vi "Example1.vi"() -> ()   [LabVIEW 2020, in "LcPictureBox.lvclass"]
uses:
  LcPictureBox.lvclass
  SmoothingMode.ctl
  Pen.ctl
  <vilib>/numeric/Random Number (Range) U64.vi
  <vilib>/numeric/Random Number (Range) DBL.vi
  <vilib>/numeric/sub_Random U32.vi
  System.Windows.Forms
panel:
  in  "PictureBox":refnum<k24>(container)
  in  "Stop":bool
  out "Updating":u32
  out "Drawing":u32
  out "error out":errorcluster
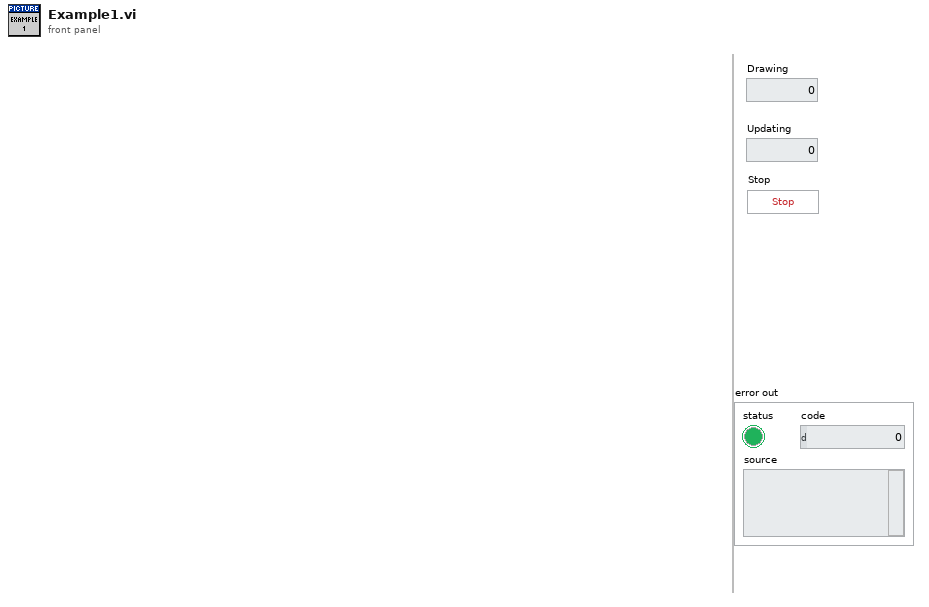
[diagram p1: front panel]
types:
  T1 = typedef "LcPictureBox.lvclass/SmoothingMode.ctl" = enum16{"None", "HighSpeed", "HighQuality", "AntiAlias"}
  T2 = typedef "LcPictureBox.lvclass/Pen.ctl" = cluster{"Width":u16, "Style":enum32{"Solid", "Dash", "Dot", "DashDot", "DashDotDot"}}
  T3 = cluster{"X":sgl, "Y":sgl, "Width":sgl, "Height":sgl}
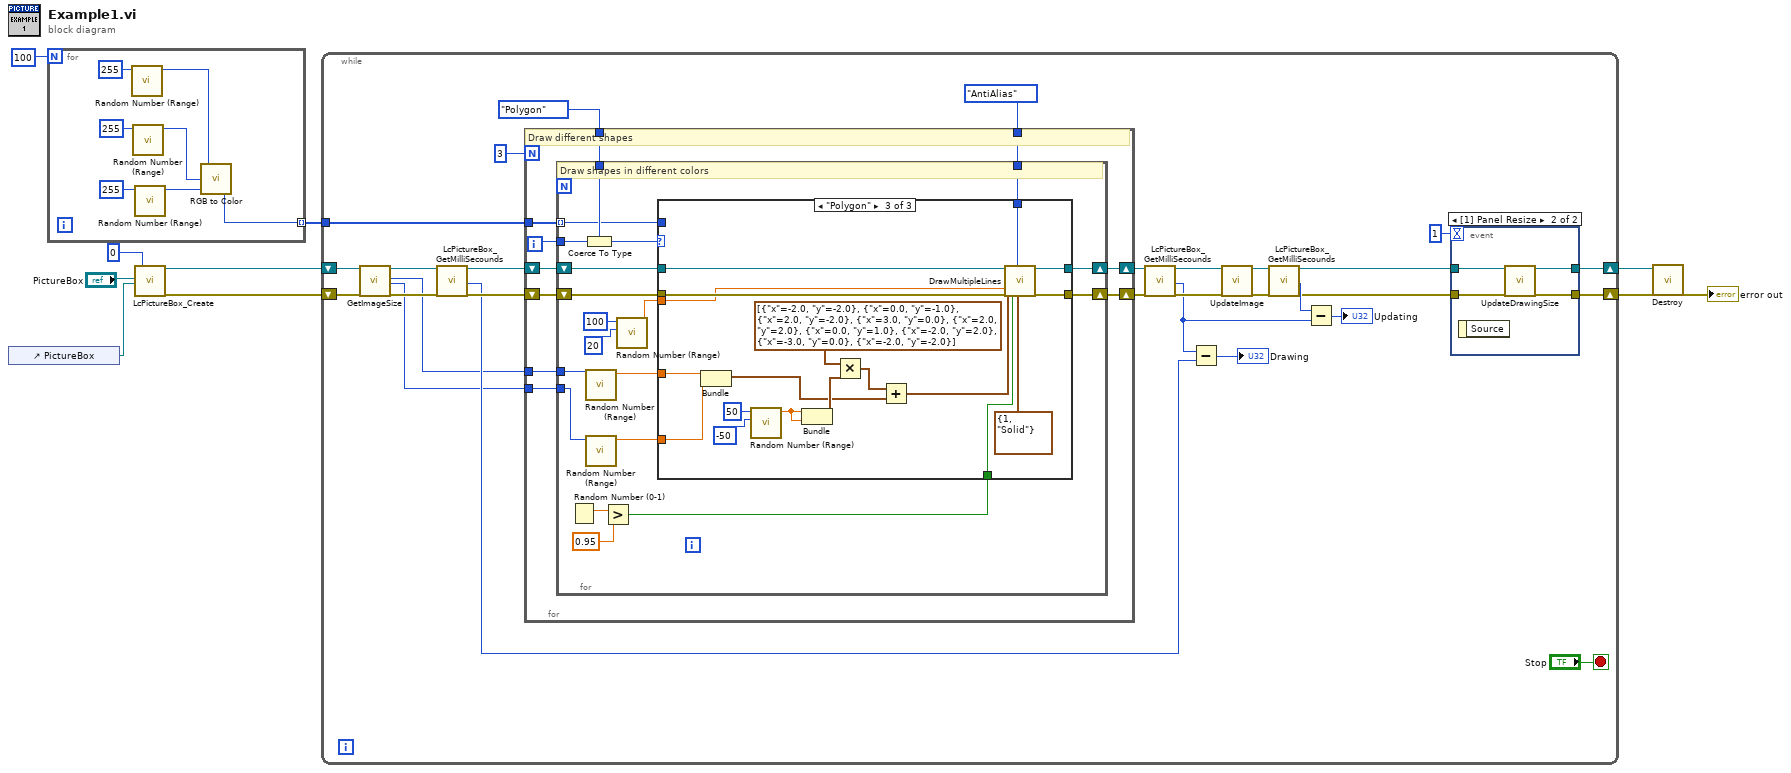
[diagram p0: block diagram]
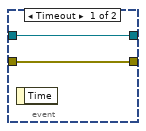
[diagram p2: hidden frame]
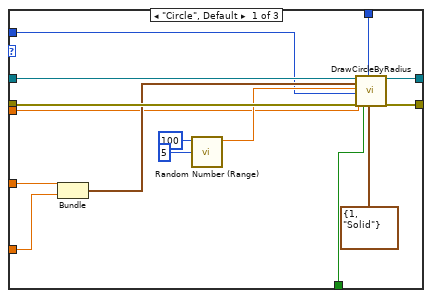
[diagram p3: hidden frame]
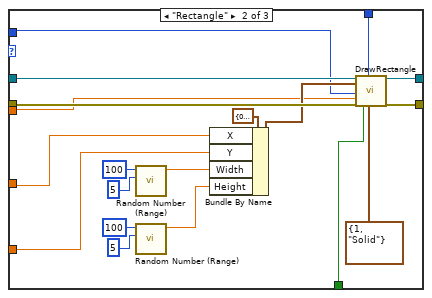
[diagram p4: hidden frame]
diagram:
  n1 = control-ref of="PictureBox"() -> (w2:refnum<vi>)
  n2 = for {
    N: 100 -> [_]
    tunnel: [w11] -> w4 mode=indexing
    n3 = call-poly <vilib>:"Random Number (Range).vi"("upper bound (100)"=u64 255) -> ("number"=w12:u64)  [unwired: 10 in]
    n4 = call-poly <vilib>:"Random Number (Range).vi"("upper bound (100)"=u64 255) -> ("number"=w13:u64)  [unwired: 10 in]
    n5 = call-poly <vilib>:"Random Number (Range).vi"("upper bound (100)"=u64 255) -> ("number"=w15:u64)  [unwired: 10 in]
    n6 = call <vilib>:"RGB to Color.vi"("B"=w15, "G"=w13, "R"=w12) -> ("Color"=w11:u32)
  }
  n7 = call "LcPictureBox_Create.vi"("PictureBox"="PictureBox", "PictureBoxActiveXReference"=w2, "CacheNumberOfPensAndColors(0)"=0 ("CacheNumberOfPensAndColors(1000)")) -> ("reference out"=w7:refnum<class "LcPictureBox.lvclass">, "Error Out"=w6:errorcluster)  [unwired: 14 in, 1 out]
  n8 = while {
    shift-right: [w25] -> w8
    shift-left: w7 -> [w23]
    shift-right: [w24] -> w10
    shift-left: w6 -> [w18]
    tunnel: w4 -> [w30]
    stop <- "Stop" stop-if-true
    n9 = call-dynamic "GetImageSize.vi"("reference in"=w23, "error in (no error)"=w18) -> ("reference out"=w22:refnum<class "LcPictureBox.lvclass">, "Width"=w20:i32, "Height"=w19:i32, "error out"=w21:errorcluster)  [unwired: 14 in]
    n10 = call "LcPictureBox_GetMilliSecounds.vi"("error in (no error)"=w21) -> ("msValue"=w29:u32, "error out"=w42:errorcluster)  [unwired: 17 in]
    n11 = for {
      N: 3 -> [_]
      tunnel: SmoothingMode."AntiAlias" ("SmoothingMode") -> [w55]
      shift-right: [w57] -> w37
      shift-left: w22 -> [w59]
      shift-right: [w58] -> w43
      shift-left: w42 -> [w56]
      tunnel: enum16{"Circle", "Rectangle", "Polygon"}."Polygon" -> [w53]
      tunnel: w20 -> [w52]
      tunnel: w19 -> [w51]
      tunnel: w30 -> [w50]
      i -> [w54]
      # "Draw different shapes"
      n12 = for {
        shift-right: [w75] -> w57
        shift-left: w59 -> [w78]
        shift-right: [w76] -> w58
        shift-left: w56 -> [w77]
        tunnel: w55 -> [w74]
        tunnel: w54 -> [w73]
        tunnel: w53 -> [w71]
        tunnel: w52 -> [w70]
        tunnel: w51 -> [w69]
        tunnel: w50 -> [w63] mode=indexing
        # "Draw shapes in different colors"
        n13 = Random Number (0-1)() -> (number: 0 to 1=w62:dbl)
        n14 = Coerce To Type(0:w73, 1:w71) -> (2:w72:enum16{"Circle", "Rectangle", "Polygon"})
        n15 = call-poly <vilib>:"Random Number (Range).vi"("upper bound (100)"=w70) -> ("number"=w68:dbl)  [unwired: 10 in]
        n16 = call-poly <vilib>:"Random Number (Range).vi"("upper bound (100)"=w69) -> ("number"=w67:dbl)  [unwired: 10 in]
        n17 = Greater?(x=w62, y=0.95) -> (0:w60:bool)
        n18 = call-poly <vilib>:"Random Number (Range).vi"("lower bound (0)"=i64 20 ("lower bound (-100)"), "upper bound (100)"=i64 100) -> ("number"=w64:dbl)  [unwired: 9 in]
        n19 = case shown="\"Polygon\"" w72 {
          tunnel: w78 -> [w93 w112 w130]
          tunnel: w77 -> [w92 w111 w129]
          tunnel: [w91 w110 w128] -> w76
          tunnel: [w90 w109 w127] -> w75
          tunnel: w74 -> [w88 w107 w125]
          tunnel: w68 -> [w87 w104 w124]
          tunnel: w67 -> [w86 w103 w123]
          tunnel: w64 -> [w81 w95 w121]
          tunnel: w63 -> [w80 w96 _]
          tunnel: w60 -> [w79 w94 w120]
          frame "Circle", Default {
            n20 = Bundle("number"=w87, "number"=w86) -> (w85:cluster{"number":dbl, "number":dbl})  [unwired: 1 in]
            n21 = call-poly <vilib>:"Random Number (Range).vi"("lower bound (0)"=i64 5 ("lower bound (-100)"), "upper bound (100)"=i64 100) -> ("number"=w82:dbl)  [unwired: 9 in]
            n22 = call-dynamic "DrawCircleByRadius.vi"("reference in"=w93, "Center"=w85, "Radius"=w82, "Color(Black)"=w80, "Alpha(100%)"=w81, "Error In"=w92, "Fill(False)"=w79, "SmoothingMode(AntiAlias)"=w88, "Pen(Width=1, Solid)"=T2 {"Width"=1, "Style"=enum."Solid"}) -> ("reference out"=w90:refnum<class "LcPictureBox.lvclass">, "Error Out"=w91:errorcluster)  [unwired: 9 in]
          }
          frame "Rectangle" {
            n23 = call-poly <vilib>:"Random Number (Range).vi"("lower bound (0)"=i64 5 ("lower bound (-100)"), "upper bound (100)"=i64 100) -> ("number"=w100:dbl)  [unwired: 9 in]
            n24 = call-poly <vilib>:"Random Number (Range).vi"("lower bound (0)"=i64 5 ("lower bound (-100)"), "upper bound (100)"=i64 100) -> ("number"=w97:dbl)  [unwired: 9 in]
            n25 = Bundle By Name(cluster=T3 {"X"=0.0, "Y"=0.0, "Width"=0.0, "Height"=0.0} ("Rectangle"), "X"=w104, "Y"=w103, "Width"=w100, "Height"=w97) -> (w105:T3)
            n26 = call-dynamic "DrawRectangle.vi"("reference in"=w112, "Rectangle"=w105, "Color(Black)"=w96, "Alpha(100%)"=w95, "Error In"=w111, "Fill(False)"=w94, "SmoothingMode(None)"=w107, "Pen(Width=1, Solid)"=T2 {"Width"=1, "Style"=enum."Solid"}) -> ("reference out"=w109:refnum<class "LcPictureBox.lvclass">, "Error Out"=w110:errorcluster)  [unwired: 10 in]
          }
          frame "Polygon" {
            n27 = Bundle("number"=w124, "number"=w123) -> (w113:cluster{"number":dbl, "number":dbl})  [unwired: 1 in]
            n28 = call-poly <vilib>:"Random Number (Range).vi"("lower bound (0)"=i64 -50 ("lower bound (-100)"), "upper bound (100)"=i64 50) -> ("number"=w117:dbl)  [unwired: 9 in]
            n29 = Bundle("number"=w117, "number"=w117) -> (w116:cluster{"number":dbl, "number":dbl})  [unwired: 1 in]
            n30 = Multiply(x=cluster{"x":dbl, "y":dbl}[] [{"x"=-2.0, "y"=-2.0}, {"x"=0.0, "y"=-1.0}, {"x"=2.0, "y"=-2.0}, {"x"=3.0, "y"=0.0}, {"x"=2.0, "y"=2.0}, {"x"=0.0, "y"=1.0}, {"x"=-2.0, "y"=2.0}, {"x"=-3.0, "y"=0.0}, {"x"=-2.0, "y"=-2.0}] ("LineEndPoints"), y=w116) -> (x*y=w115:cluster{dbl, dbl}[])
            n31 = Add(x=w115, y=w113) -> (x+y=w122:cluster{dbl, dbl}[])
            n32 = call-dynamic "DrawMultipleLines.vi"("reference in"=w130, "LineEndPoints"=w122, "Alpha(100%)"=w121, "Error In"=w129, "Fill(False)"=w120, "SmoothingMode(AntiAlias)"=w125, "Pen(Width=1, Solid)"=T2 {"Width"=1, "Style"=enum."Solid"}) -> ("reference out"=w127:refnum<class "LcPictureBox.lvclass">, "Error Out"=w128:errorcluster)  [unwired: 11 in]
          }
        }
      }
    }
    n33 = call "LcPictureBox_GetMilliSecounds.vi"("error in (no error)"=w43) -> ("msValue"=w33:u32, "error out"=w38:errorcluster)  [unwired: 17 in]
    n34 = Subtract(x=w33, y=w29) -> (x-y=→"Drawing":u32)
    n35 = call-dynamic "UpdateImage.vi"("reference in"=w37, "Error In"=w38) -> ("reference out"=w28:refnum<class "LcPictureBox.lvclass">, "Error Out"=w36:errorcluster)  [unwired: 14 in, 2 out]
    n36 = call "LcPictureBox_GetMilliSecounds.vi"("error in (no error)"=w36) -> ("msValue"=w34:u32, "error out"=w26:errorcluster)  [unwired: 17 in]
    n37 = Subtract(x=w34, y=w33) -> (x-y=→"Updating":u32)
    n38 = event shown="[1] Panel Resize" {
      selector: _ -> [_ _]
      dyn-events: _ -> [_ _]
      timeout: 1 -> [_ _]
      tunnel: w28 -> [w45 w49]
      tunnel: w26 -> [w44 w48]
      tunnel: [w45 w47] -> w25
      tunnel: [w44 w46] -> w24
      event Timeout {
        n39 = event-data() -> ()  [unwired: 1 in, 1 out]
      }
      event Panel Resize {
        n40 = event-data() -> ()  [unwired: 1 in, 1 out]
        n41 = call-dynamic "UpdateDrawingSize.vi"("reference in"=w49, "Error In"=w48) -> ("reference out"=w47:refnum<class "LcPictureBox.lvclass">, "Error Out"=w46:errorcluster)  [unwired: 16 in]
      }
    }
  }
  n42 = call-dynamic "Destroy.vi"("reference in"=w8, "Error In"=w10) -> ("Error Out"=→"error out":errorcluster)  [unwired: 16 in, 1 out]
